vi "main.vi"() -> ()   [LabVIEW 2015]
uses:
  USB Template (LV 8.6)/Boiler/Controls/Boiler Controls.ctl
  USB Template (LV 8.6)/Boiler/Controls/Boiler Simulation Controls.ctl
  USB Template (LV 8.6)/Boiler/Controls/Boiler Status Indicators.ctl
  Controls/state.ctl
  Controls/timer status.ctl
  <vilib>/Utility/file.llb/Write Delimited Spreadsheet (string).vi
panel:
  out "error out":errorcluster
  in  "error in":errorcluster
  in  "stop":bool
  out "Boiler Status Indicators":T1 {"Time Count" format="%.2g"}
  in  "Boiler Simulation Controls":T2 {"Flame Sensor Value (%)" min=0.0 max=100.0 scale=0.0..100.0}
  in  "Boiler Controls":T3 {"Fuel Valve Position" min=0.0 max=100.0 scale=0.0..100.0 scale format="%.2f"}
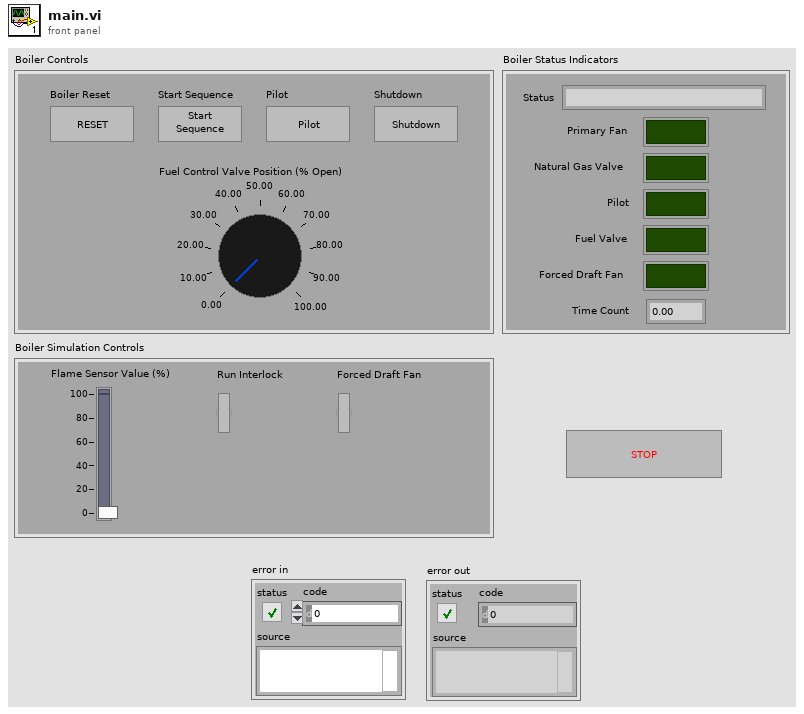
[diagram p1: front panel]
types:
  T1 = typedef "Boiler Status Indicators.ctl" = cluster{"Status":string, "Primary Fan":bool, "Natural Gas Valve":bool, "Pilot":bool, "Fuel Valve":bool, "Forced Draft Fan":bool, "Time Count":dbl}
  T2 = typedef "Boiler Simulation Controls.ctl" = cluster{"Flame Sensor Value (%)":dbl, "Run Interlock":bool, "Forced Draft Fan":bool}
  T3 = typedef "Boiler Controls.ctl" = cluster{"Boiler Reset":bool, "Start Sequence":bool, "Pilot":bool, "Shutdown":bool, "Fuel Valve Position":dbl}
  T4 = typedef "state.ctl" = enum16{"Initialize", "Idle", "Reset Lockout", "Pre-Purge", "Pre-Purge 2", "Ignition", "Prove Pilot", "Run", "Start", "Shutdown&Purge", "Error", "Exit"}
  T5 = typedef "timer status.ctl" = enum16{"Stop", "Start"}
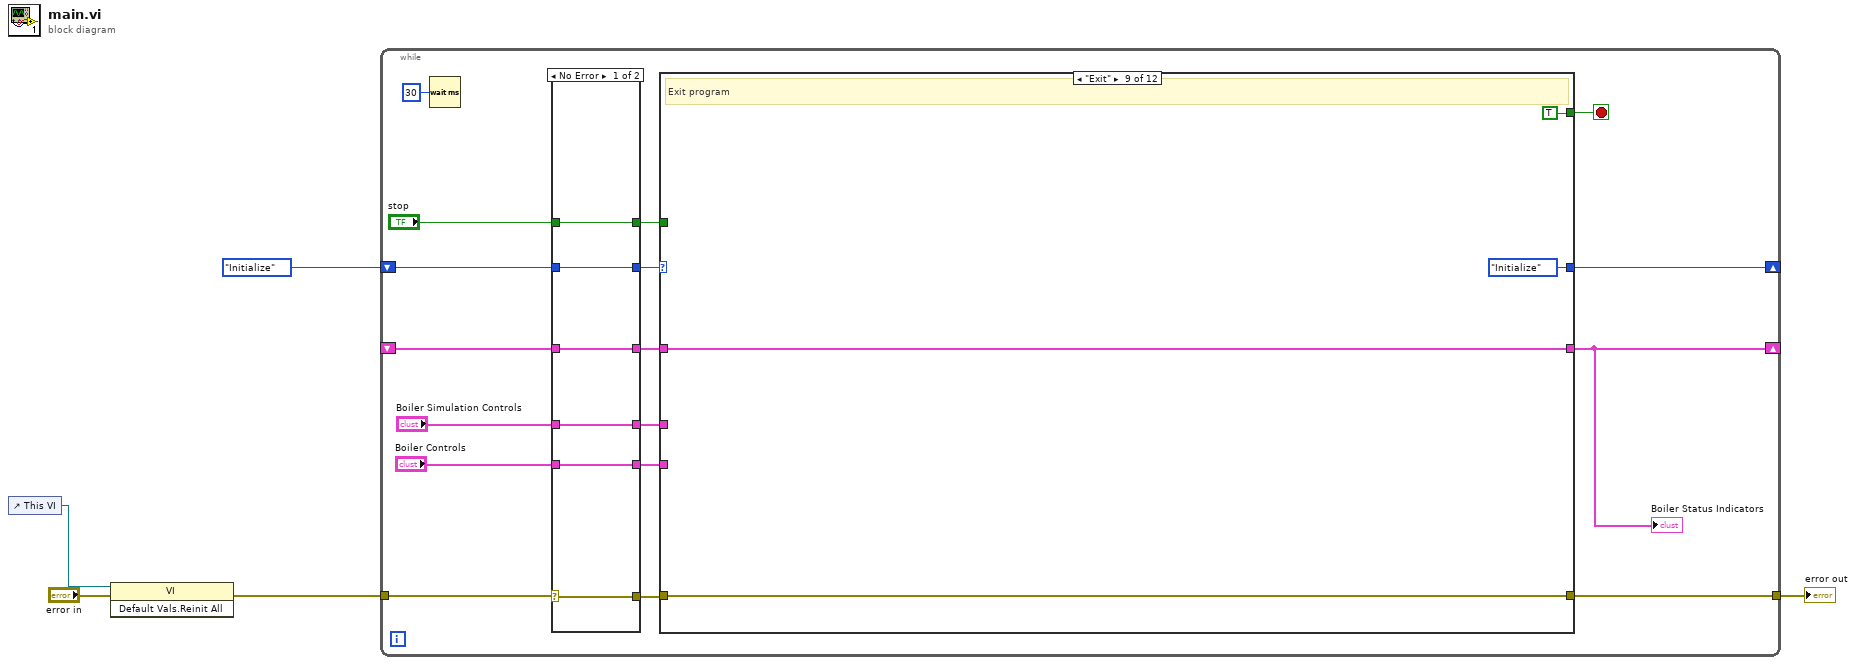
[diagram p0: block diagram]
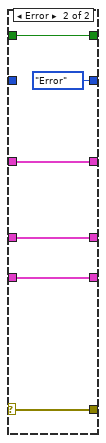
[diagram p2: hidden frame]
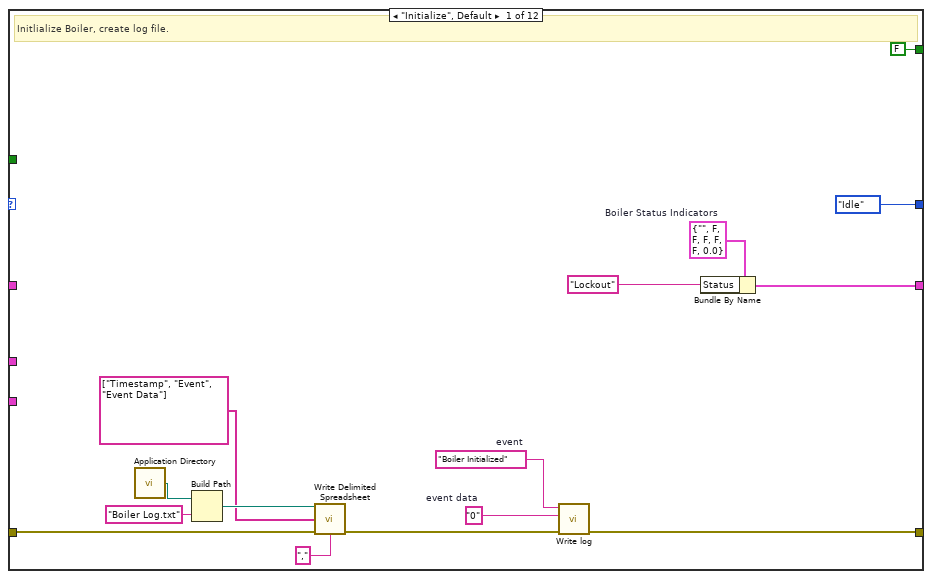
[diagram p3: hidden frame]
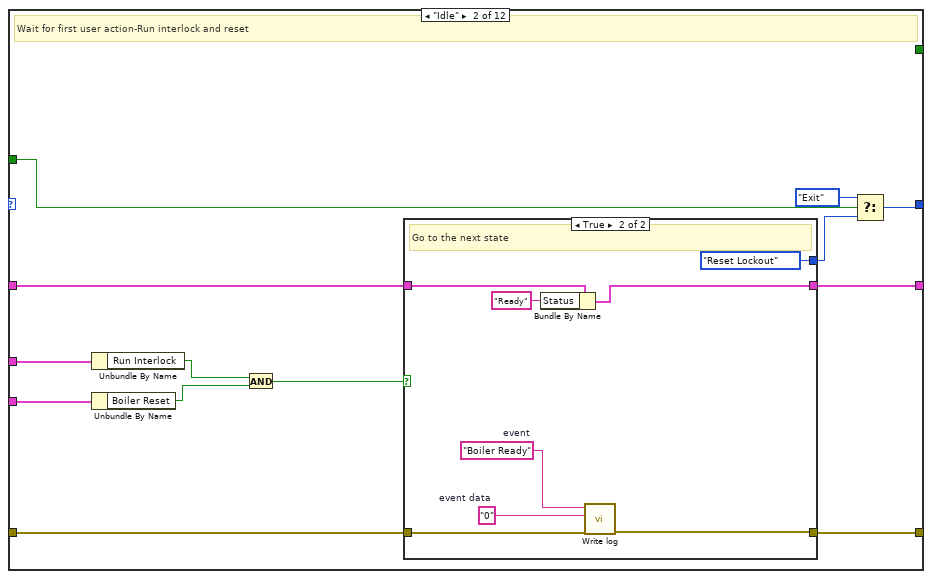
[diagram p4: hidden frame]
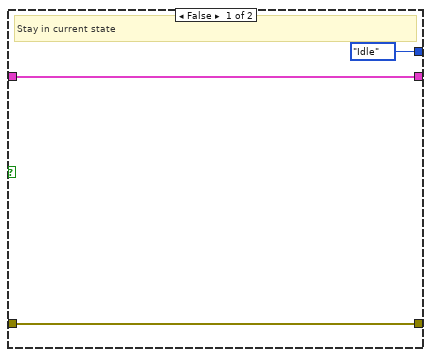
[diagram p5: hidden frame]
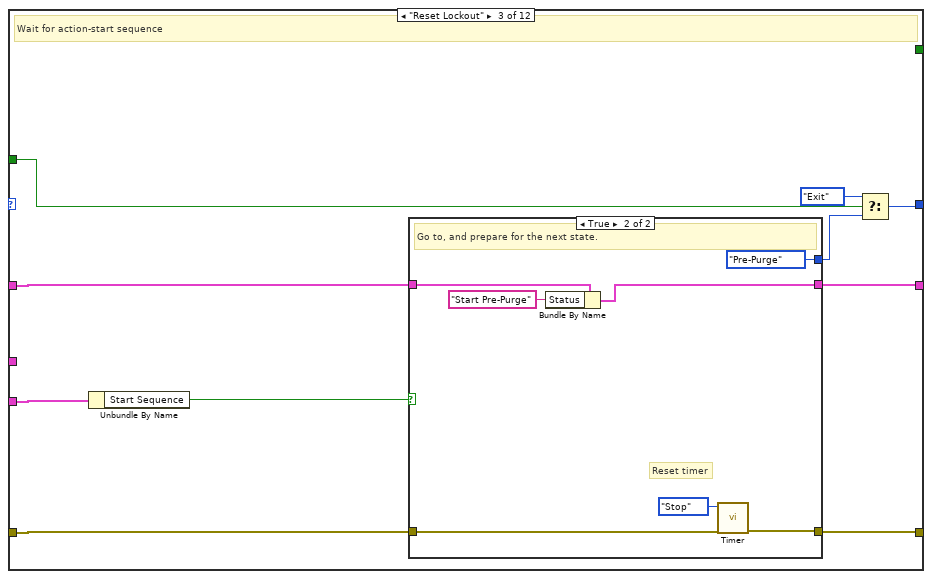
[diagram p6: hidden frame]
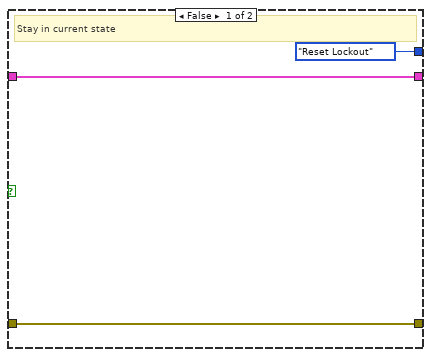
[diagram p7: hidden frame]
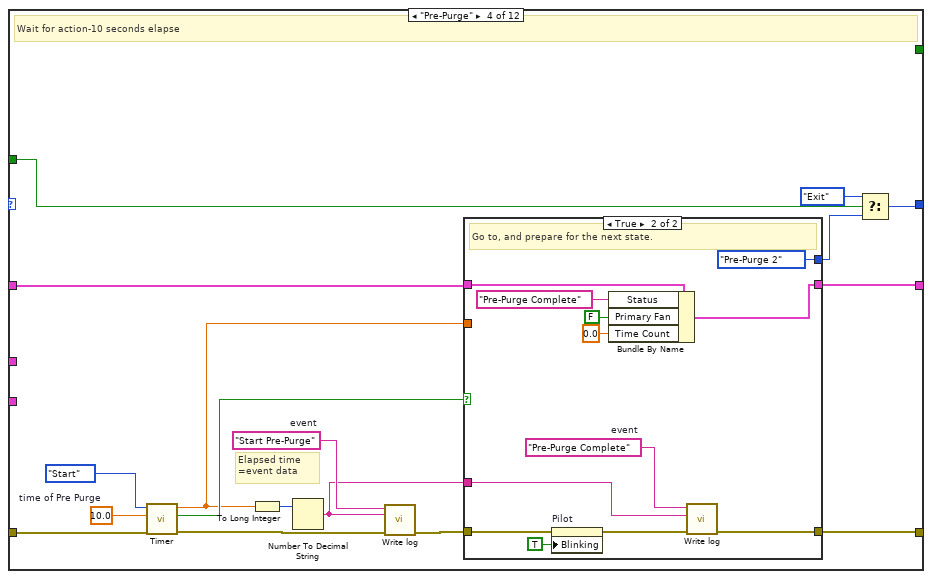
[diagram p8: hidden frame]
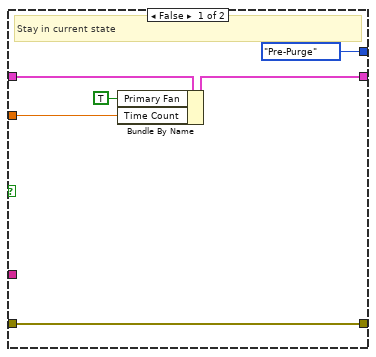
[diagram p9: hidden frame]
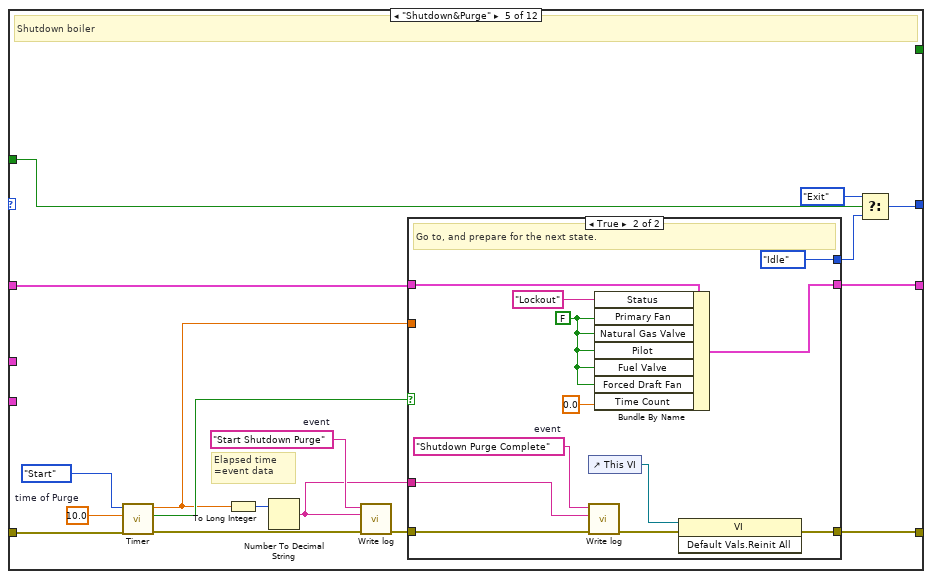
[diagram p10: hidden frame]
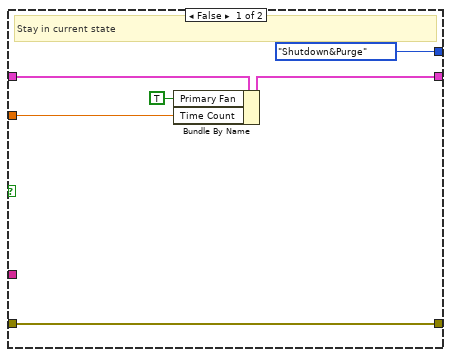
[diagram p11: hidden frame]
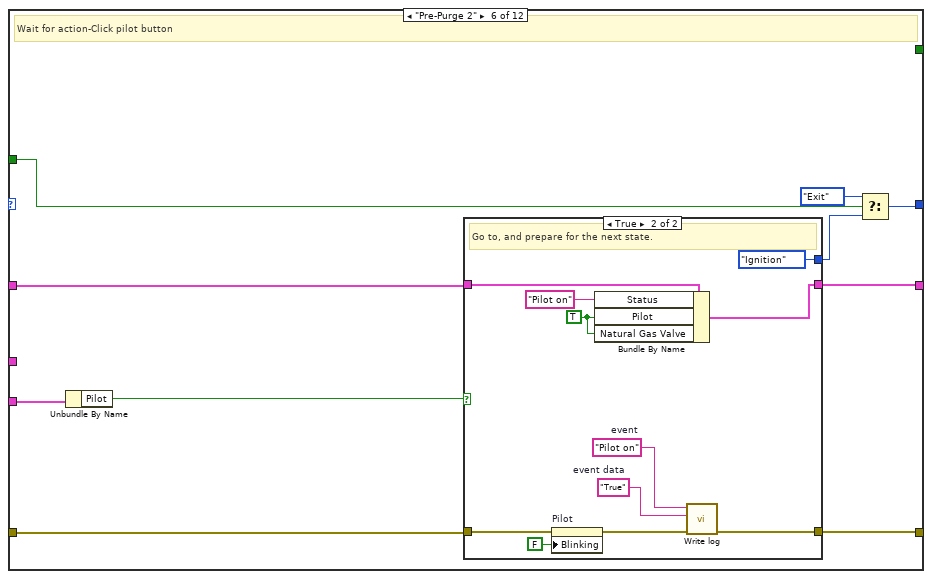
[diagram p12: hidden frame]
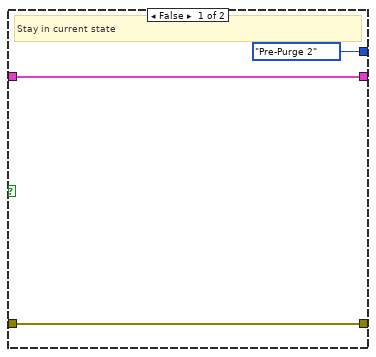
[diagram p13: hidden frame]
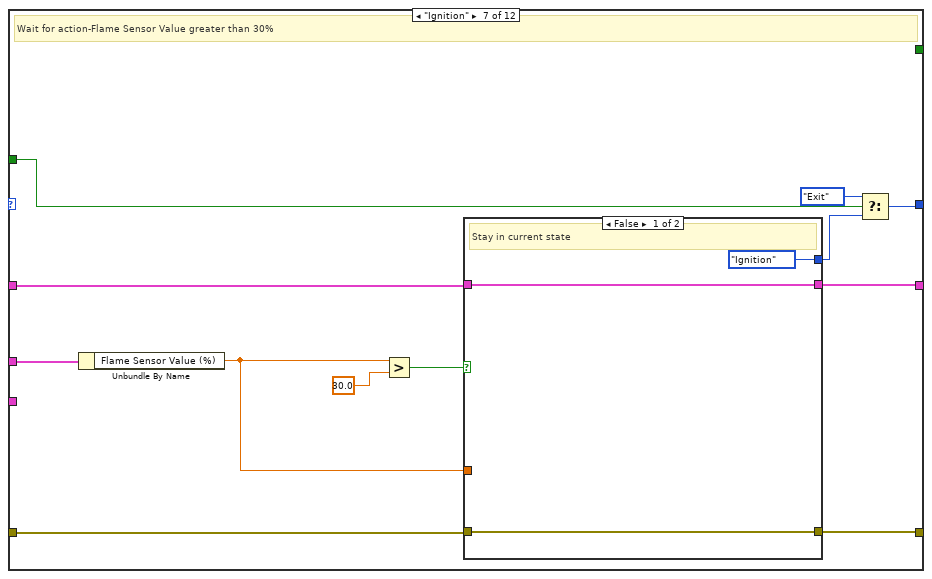
[diagram p14: hidden frame]
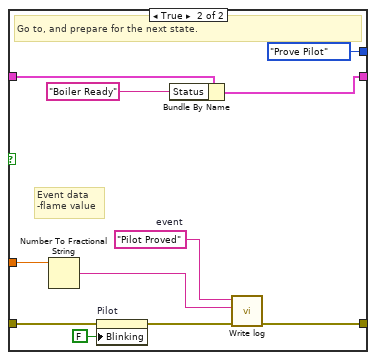
[diagram p15: hidden frame]
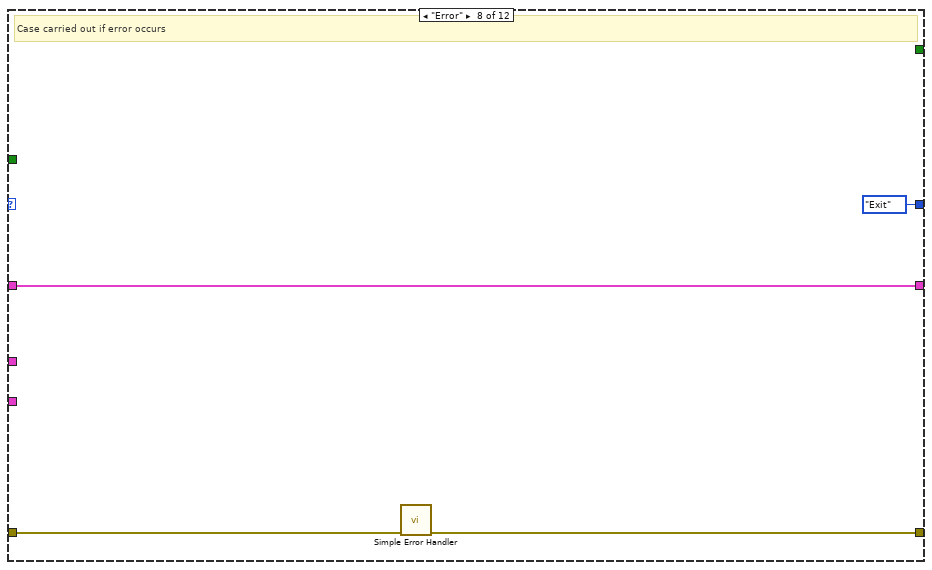
[diagram p16: hidden frame]
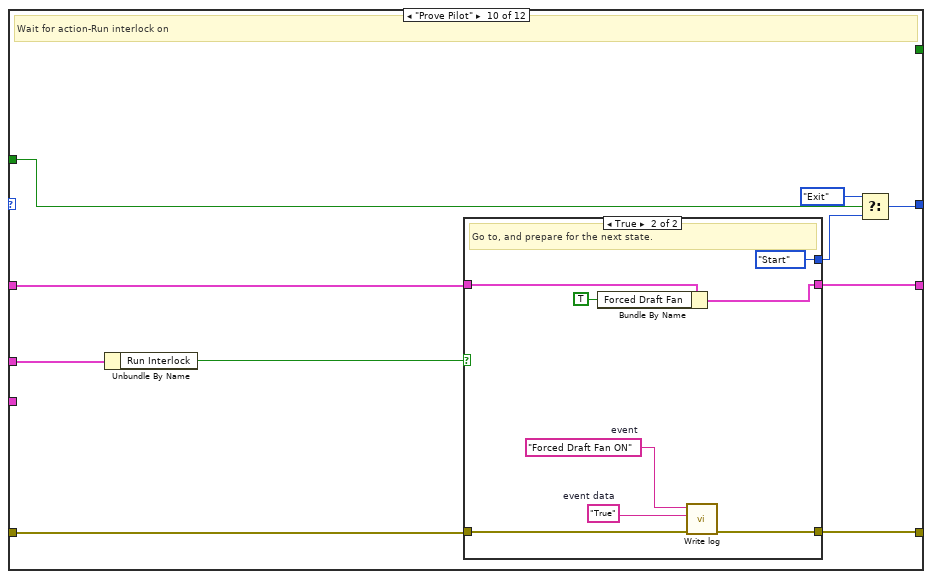
[diagram p17: hidden frame]
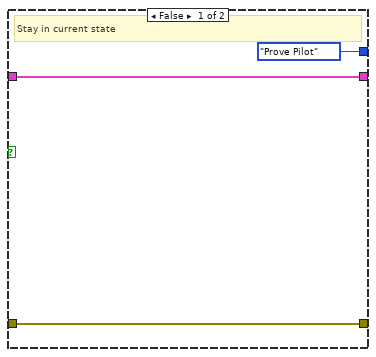
[diagram p18: hidden frame]
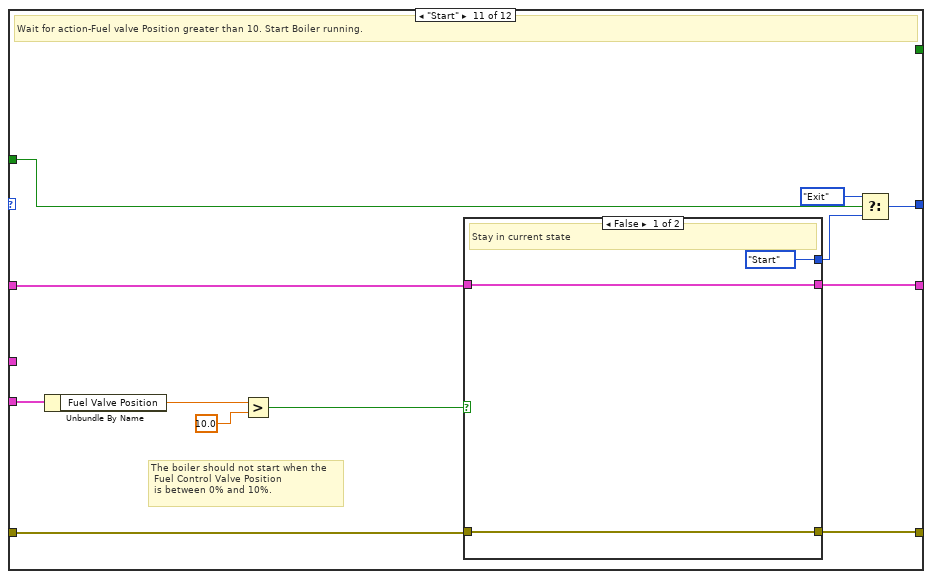
[diagram p19: hidden frame]
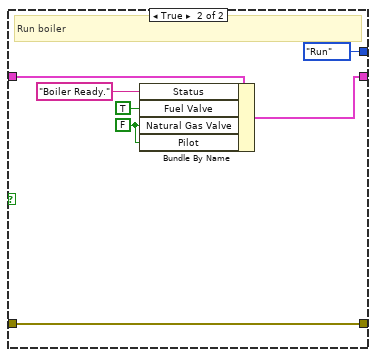
[diagram p20: hidden frame]
diagram:
  n1 = control-ref of="This VI"() -> (w3:refnum<vi>)
  n2 = invoke class="VI" method="Default Vals.Reinit All"(reference=w3, error in="error in") -> (error out=w2:errorcluster)  [unwired: 1 in, 2 out]
  n3 = while {
    tunnel: w2 -> [w17]
    tunnel: [w22] -> w4
    shift-right: [w20] -> _
    shift-left: _ -> [w6]
    shift-right: [w19] -> _
    shift-left: state."Initialize" ("state") -> [w11]
    stop <- w21 stop-if-true
    n4 = Wait (ms)(milliseconds to wait=u32 30) -> ()  [unwired: 1 out]
    n5 = case shown="No Error" w17 {
      selector: w17 -> [w28 w30]
      tunnel: [w28 w30] -> w16
      tunnel: [w27 w31] -> w15
      tunnel: "Boiler Controls" -> [w27 w31]
      tunnel: [w26 w32] -> w13
      tunnel: "Boiler Simulation Controls" -> [w26 w32]
      tunnel: w11 -> [w25 _]
      tunnel: [w25 state."Error" ("state")] -> w10
      tunnel: "stop" -> [w24 w33]
      tunnel: [w24 w33] -> w8
      tunnel: [w23 w29] -> w7
      tunnel: w6 -> [w23 w29]
      frame No Error {
      }
      frame Error {
      }
    }
    n6 = case shown="\"Exit\"" w10 {
      tunnel: w16 -> [w37 w62 w81 w102 w137 w166 w192 w216 w218 w224 w247 w269]
      tunnel: [w45 w61 w77 w106 w141 w169 w195 w215 w218 w227 w250 w273] -> w22
      tunnel: [FALSE _ _ _ _ _ _ _ TRUE _ _ _] -> w21
      tunnel: [w46 w54 w76 w105 w140 w168 w194 w214 w219 w226 w249 w272] -> w20
      tunnel: [state."Idle" ("state") w50 w75 w104 w139 w167 w193 state."Exit" ("state") state."Initialize" ("state") w225 w248 w271] -> w19
      tunnel: w13 -> [_ w60 _ _ _ _ w191 _ _ w223 _ w266]
      tunnel: w15 -> [_ w59 w80 _ _ w165 _ _ _ _ w243 w265]
      tunnel: w7 -> [_ w55 w79 w108 w143 w171 w197 w214 w219 w229 w252 w275]
      tunnel: w8 -> [_ w52 w78 w107 w142 w170 w196 _ _ w228 w251 w274]
      frame "Initialize", Default {
        w43 = "0"  # event data
        w44 = "Boiler Initialized"  # event
        w48 = T1 {"Status"="", "Primary Fan"=FALSE, "Natural Gas Valve"=FALSE, "Pilot"=FALSE, "Fuel Valve"=FALSE, "Forced Draft Fan"=FALSE, "Time Count"=0.0}  # Boiler Status Indicators
        # "Initlialize Boiler, create log file."
        n7 = call <vilib>:"Application Directory.vi"() -> ("Application Directory"=w41:path)
        n8 = Build Path(base path=w41, name or relative path="Boiler Log.txt") -> (appended path=w39:path)
        n9 = call-poly <vilib>:"Write Delimited Spreadsheet.vi"("file path (dialog if empty)"=w39, "1D data"=string[] ["Timestamp", "Event", "Event Data"], "error in (no error)"=w37, "delimiter (\\t)"="," ("delimiter (\\t)")) -> ("error out"=w36:errorcluster)  [unwired: 10 in, 1 out]
        n10 = call "Write log.vi"("error in (no error)"=w36, "event data"=w43, "event"=w44) -> ("error out"=w45:errorcluster)  [unwired: 8 in]
        n11 = Bundle By Name(cluster=w48, "Status"="Lockout") -> (w46:T1)
      }
      frame "Idle" {
        # "Wait for first user action-Run interlock and reset"
        n12 = Unbundle By Name(w60) -> ("Run Interlock"=w58:bool)
        n13 = Unbundle By Name(w59) -> ("Boiler Reset"=w57:bool)
        n14 = And(x=w58, y=w57) -> (x .and. y?=w56:bool)
        n15 = case shown="True" w56 {
          tunnel: w62 -> [w65 w70]
          tunnel: [w65 w66] -> w61
          tunnel: w55 -> [w64 w73]
          tunnel: [w64 w71] -> w54
          tunnel: [state."Idle" ("state") state."Reset Lockout" ("state")] -> w53
          frame False {
            # "Stay in current state"
          }
          frame True {
            w68 = "0"  # event data
            w69 = "Boiler Ready"  # event
            # "Go to the next state"
            n16 = Bundle By Name(cluster=w73, "Status"="Ready") -> (w71:T1)
            n17 = call "Write log.vi"("error in (no error)"=w70, "event data"=w68, "event"=w69) -> ("error out"=w66:errorcluster)  [unwired: 8 in]
          }
        }
        n18 = Select(t=state."Exit", s=w52, f=w53) -> (s? t:f=w50:T4)
      }
      frame "Reset Lockout" {
        # "Wait for action-start sequence"
        n19 = Unbundle By Name(w80) -> ("Start Sequence"=w74:bool)
        n20 = case shown="True" w74 {
          tunnel: w81 -> [w86 w87]
          tunnel: [w86 w89] -> w77
          tunnel: w79 -> [w85 w93]
          tunnel: [w85 w91] -> w76
          tunnel: [state."Reset Lockout" ("state") state."Pre-Purge" ("state")] -> w82
          frame False {
            # "Stay in current state"
          }
          frame True {
            # "Reset timer"
            # "Go to, and prepare for the next state."
            n21 = Bundle By Name(cluster=w93, "Status"="Start Pre-Purge") -> (w91:T1)
            n22 = call "Timer.vi"("error in"=w87, "timer state"=timer_status."Stop") -> ("error out"=w89:errorcluster)  [unwired: 7 in, 2 out]
          }
        }
        n23 = Select(t=state."Exit", s=w78, f=w82) -> (s? t:f=w75:T4)
      }
      frame "Pre-Purge" {
        w95 = "Start Pre-Purge"  # event
        w99 = 10.0  # time of Pre Purge
        # "Elapsed time\n=event data"
        # "Wait for action-10 seconds elapse"
        n24 = call "Timer.vi"("error in"=w102, "limit"=w99, "timer state"=timer_status."Start") -> ("error out"=w101:errorcluster, "limit reached"=w98:bool, "elapsed"=w97:dbl)  [unwired: 6 in]
        n25 = To Long Integer(number=w97) -> (32bit integer=w96:i32)
        n26 = Number To Decimal String(number=w96) -> (decimal integer string=w94:string)  [unwired: 1 in]
        n27 = call "Write log.vi"("error in (no error)"=w101, "event data"=w94, "event"=w95) -> ("error out"=w103:errorcluster)  [unwired: 8 in]
        n28 = case shown="True" w98 {
          tunnel: w103 -> [w116 w122]
          tunnel: [w116 w119] -> w106
          tunnel: w108 -> [w114 w128]
          tunnel: [w113 w126] -> w105
          tunnel: [state."Pre-Purge" ("state") state."Pre-Purge 2" ("state")] -> w109
          tunnel: w97 -> [w111 _]
          tunnel: w94 -> [_ w118]
          frame False {
            # "Stay in current state"
            n29 = Bundle By Name(cluster=w114, "Primary Fan"=TRUE, "Time Count"=w111) -> (w113:T1)
          }
          frame True {
            w117 = "Pre-Purge Complete"  # event
            # "Go to, and prepare for the next state."
            n30 = property on="Pilot" class="Bool (strict)"(error in=w122, "Blinking"=TRUE) -> (error out=w120:errorcluster)  [unwired: 1 in, 1 out]
            n31 = Bundle By Name(cluster=w128, "Status"="Pre-Purge Complete", "Primary Fan"=FALSE, "Time Count"=0.0) -> (w126:T1)
            n32 = call "Write log.vi"("error in (no error)"=w120, "event data"=w118, "event"=w117) -> ("error out"=w119:errorcluster)  [unwired: 8 in]
          }
        }
        n33 = Select(t=state."Exit", s=w107, f=w109) -> (s? t:f=w104:T4)
      }
      frame "Shutdown&Purge" {
        w130 = "Start Shutdown Purge"  # event
        w134 = 10.0  # time of Purge
        # "Elapsed time\n=event data"
        # "Shutdown boiler"
        n34 = call "Timer.vi"("error in"=w137, "limit"=w134, "timer state"=timer_status."Start") -> ("error out"=w136:errorcluster, "limit reached"=w133:bool, "elapsed"=w132:dbl)  [unwired: 6 in]
        n35 = To Long Integer(number=w132) -> (32bit integer=w131:i32)
        n36 = Number To Decimal String(number=w131) -> (decimal integer string=w129:string)  [unwired: 1 in]
        n37 = call "Write log.vi"("error in (no error)"=w136, "event data"=w129, "event"=w130) -> ("error out"=w138:errorcluster)  [unwired: 8 in]
        n38 = case shown="True" w133 {
          tunnel: w138 -> [w146 w157]
          tunnel: [w146 w152] -> w141
          tunnel: w143 -> [w150 w163]
          tunnel: [w149 w161] -> w140
          tunnel: [state."Shutdown&Purge" ("state") state."Idle" ("state")] -> w144
          tunnel: w132 -> [w147 _]
          tunnel: w129 -> [_ w159]
          frame False {
            # "Stay in current state"
            n39 = Bundle By Name(cluster=w150, "Primary Fan"=TRUE, "Time Count"=w147) -> (w149:T1)
          }
          frame True {
            w158 = "Shutdown Purge Complete"  # event
            w155 = FALSE ("Primary Fan")
            # "Go to, and prepare for the next state."
            n40 = control-ref of="This VI"() -> (w154:refnum<vi>)
            n41 = call "Write log.vi"("error in (no error)"=w157, "event data"=w159, "event"=w158) -> ("error out"=w153:errorcluster)  [unwired: 8 in]
            n42 = Bundle By Name(cluster=w163, "Status"="Lockout", "Primary Fan"=w155, "Natural Gas Valve"=w155, "Pilot"=w155, "Fuel Valve"=w155, "Forced Draft Fan"=w155, "Time Count"=0.0) -> (w161:T1)
            n43 = invoke class="VI" method="Default Vals.Reinit All"(reference=w154, error in=w153) -> (error out=w152:errorcluster)  [unwired: 1 in, 2 out]
          }
        }
        n44 = Select(t=state."Exit", s=w142, f=w144) -> (s? t:f=w139:T4)
      }
      frame "Pre-Purge 2" {
        # "Wait for action-Click pilot button"
        n45 = Unbundle By Name(w165) -> ("Pilot"=w164:bool)
        n46 = case shown="True" w164 {
          tunnel: w166 -> [w176 w183]
          tunnel: [w176 w180] -> w169
          tunnel: w171 -> [w174 w187]
          tunnel: [w174 w185] -> w168
          tunnel: [state."Pre-Purge 2" ("state") state."Ignition" ("state")] -> w172
          frame False {
            # "Stay in current state"
          }
          frame True {
            w177 = "True"  # event data
            w179 = "Pilot on"  # event
            w178 = TRUE ("Primary Fan")
            # "Go to, and prepare for the next state."
            n47 = property on="Pilot" class="Bool (strict)"(error in=w183, "Blinking"=FALSE) -> (error out=w181:errorcluster)  [unwired: 1 in, 1 out]
            n48 = Bundle By Name(cluster=w187, "Status"="Pilot on", "Pilot"=w178, "Natural Gas Valve"=w178) -> (w185:T1)
            n49 = call "Write log.vi"("error in (no error)"=w181, "event data"=w177, "event"=w179) -> ("error out"=w180:errorcluster)  [unwired: 8 in]
          }
        }
        n50 = Select(t=state."Exit", s=w170, f=w172) -> (s? t:f=w167:T4)
      }
      frame "Ignition" {
        # "Wait for action-Flame Sensor Value greater than 30%"
        n51 = Unbundle By Name(w191) -> ("Flame Sensor Value (%)"=w188:dbl)
        n52 = Greater?(x=w188, y=30.0) -> (0:w189:bool)
        n53 = case shown="False" w189 {
          tunnel: w192 -> [w202 w209]
          tunnel: [w202 w206] -> w195
          tunnel: w197 -> [w200 w213]
          tunnel: [w200 w211] -> w194
          tunnel: [state."Ignition" ("state") state."Prove Pilot" ("state")] -> w198
          tunnel: w188 -> [_ w204]
          frame False {
            # "Stay in current state"
          }
          frame True {
            w205 = "Pilot Proved"  # event
            # "Event data\n-flame value"
            # "Go to, and prepare for the next state."
            n54 = Number To Fractional String(number=w204) -> (F-format string=w203:string)  [unwired: 3 in]
            n55 = property on="Pilot" class="Bool (strict)"(error in=w209, "Blinking"=FALSE) -> (error out=w207:errorcluster)  [unwired: 1 in, 1 out]
            n56 = Bundle By Name(cluster=w213, "Status"="Boiler Ready") -> (w211:T1)
            n57 = call "Write log.vi"("error in (no error)"=w207, "event data"=w203, "event"=w205) -> ("error out"=w206:errorcluster)  [unwired: 8 in]
          }
        }
        n58 = Select(t=state."Exit", s=w196, f=w198) -> (s? t:f=w193:T4)
      }
      frame "Error" {
        # "Case carried out if error occurs"
        n59 = call <vilib>:"Simple Error Handler.vi"("error in (no error)"=w216) -> ("error out"=w215:errorcluster)  [unwired: 4 in, 4 out]
      }
      frame "Exit" {
        # "Exit program"
      }
      frame "Prove Pilot" {
        # "Wait for action-Run interlock on"
        n60 = Unbundle By Name(w223) -> ("Run Interlock"=w222:bool)
        n61 = case shown="True" w222 {
          tunnel: w224 -> [w234 w235]
          tunnel: [w234 w239] -> w227
          tunnel: w229 -> [w232 w242]
          tunnel: [w232 w241] -> w226
          tunnel: [state."Prove Pilot" ("state") state."Start" ("state")] -> w230
          frame False {
            # "Stay in current state"
          }
          frame True {
            w236 = "True"  # event data
            w238 = "Forced Draft Fan ON"  # event
            # "Go to, and prepare for the next state."
            n62 = Bundle By Name(cluster=w242, "Forced Draft Fan"=TRUE) -> (w241:T1)
            n63 = call "Write log.vi"("error in (no error)"=w235, "event data"=w236, "event"=w238) -> ("error out"=w239:errorcluster)  [unwired: 8 in]
          }
        }
        n64 = Select(t=state."Exit", s=w228, f=w230) -> (s? t:f=w225:T4)
      }
      frame "Start" {
        # "The boiler should not start when the\n Fuel Control Valve Position\n is between 0% and 10%."
        # "Wait for action-Fuel valve Position greater than 10. Start Boiler running."
        n65 = Unbundle By Name(w243) -> ("Fuel Valve Position"=w244:dbl)
        n66 = Greater?(x=w244, y=10.0) -> (0:w245:bool)
        n67 = case shown="False" w245 {
          tunnel: w247 -> [w257 w258]
          tunnel: [w257 w258] -> w250
          tunnel: w252 -> [w255 w264]
          tunnel: [w255 w263] -> w249
          tunnel: [state."Start" ("state") state."Run" ("state")] -> w253
          frame False {
            # "Stay in current state"
          }
          frame True {
            w259 = FALSE ("Natural Gas Valve")
            # "Run boiler"
            n68 = Bundle By Name(cluster=w264, "Status"="Boiler Ready.", "Fuel Valve"=TRUE, "Natural Gas Valve"=w259, "Pilot"=w259) -> (w263:T1)
          }
        }
        n69 = Select(t=state."Exit", s=w251, f=w253) -> (s? t:f=w248:T4)
      }
      frame "Run" {
        # "Boiler is running"
        n70 = Unbundle By Name(w265) -> ("Fuel Valve Position"=w270:dbl)
        n71 = call "Shutdown.vi"("error in"=w269, "Boiler Controls"=w265, "Boiler Simulation Controls"=w266) -> ("error out"=w267:errorcluster, "shutdown"=w268:bool)  [unwired: 7 in]
        n72 = case shown="False" w268 {
          tunnel: w267 -> [w283 w296]
          tunnel: [w285 w295] -> w273
          tunnel: w275 -> [w288 w293]
          tunnel: [w287 w292] -> w272
          tunnel: [state."Run" ("state") state."Shutdown&Purge" ("state")] -> w276
          tunnel: w270 -> [w279 _]
          frame False {
            w280 = FALSE ("Natural Gas Valve")
            w284 = "Boiler Running"  # event
            # "Event data\n-fuel valve value"
            # "Run boiler"
            n73 = Number To Fractional String(number=w279) -> (F-format string=w278:string)  [unwired: 3 in]
            n74 = Bundle By Name(cluster=w288, "Status"="Boiler Running", "Fuel Valve"=TRUE, "Natural Gas Valve"=w280, "Pilot"=w280) -> (w287:T1)
            n75 = call "Write log.vi"("error in (no error)"=w283, "event data"=w278, "event"=w284) -> ("error out"=w285:errorcluster)  [unwired: 8 in]
          }
          frame True {
            # "Reset timer"
            # "Stay in current state"
            n76 = Bundle By Name(cluster=w293, "Status"="Purge", "Primary Fan"=TRUE, "Fuel Valve"=FALSE) -> (w292:T1)
            n77 = call "Timer.vi"("error in"=w296, "timer state"=timer_status."Stop") -> ("error out"=w295:errorcluster)  [unwired: 7 in, 2 out]
          }
        }
        n78 = Select(t=state."Exit", s=w274, f=w276) -> (s? t:f=w271:T4)
      }
    }
    "Boiler Status Indicators" <- w20
  }
  "error out" <- w4
